vi "Collect information from UI to run measurement.vi"(8 "error in (no error)":errorcluster, 11 "Measurement UI in":refnum<class "Measurement UI.lvclass">) -> (0 "error out":errorcluster, 1 "Show UI?":bool, 2 "Device Names":string[](array[string]), 3 "Measurement UI out":refnum<class "Measurement UI.lvclass">, 4 "String":string, 5 "Measurement Name":string, 6 "Run continuously?":bool, 7 "Iterations":i32)   [LabVIEW 2017, in "Measurement UI.lvlib" / "Measurement UI.lvclass"]
uses:
  Measurement UI.lvclass
  Measurement UI.lvclass/Measurement UI.ctl
  Accessors/Read Measurement.vi
  Accessors/Read Power Supply.vi
  Accessors/Read Digitizer.vi
  Accessors/Read Function Generator.vi
  Read Multimeter.vi
  Accessors/Read Show FP_.vi
  Read Run Indefinitely.vi
  Accessors/Read Step Iterations.vi
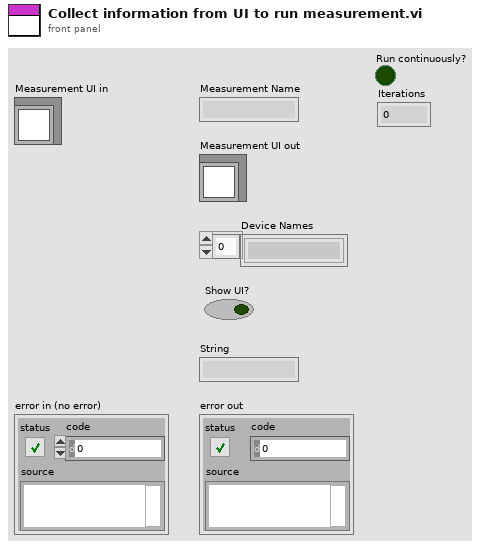
[diagram p1: front panel]
types:
  T1 = enum8{"Enabled", "Disabled", "Disabled and Grayed Out"}
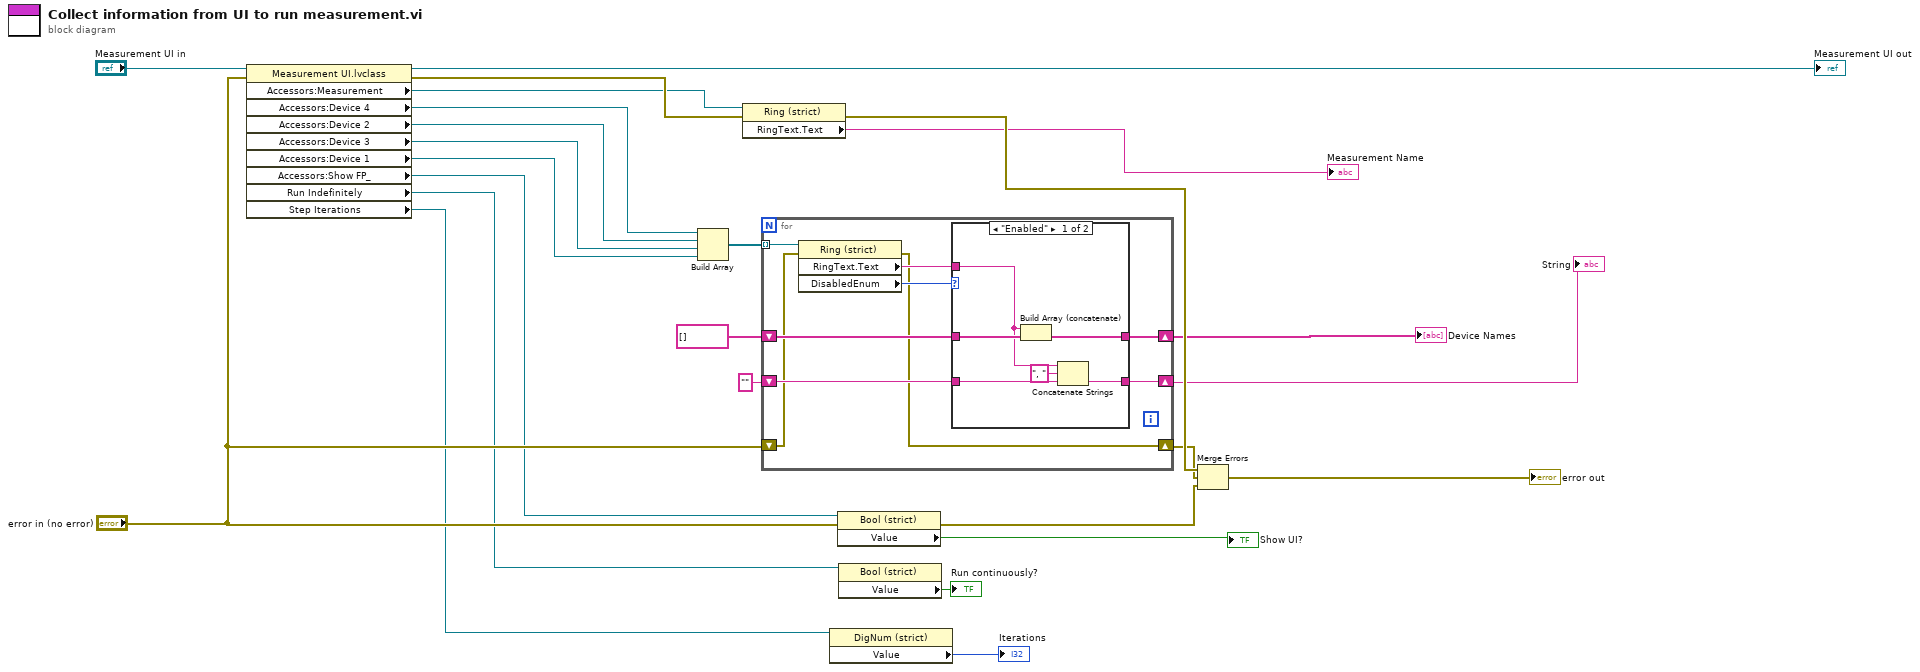
[diagram p0: block diagram]
diagram:
  n1 = property class="Measurement UI.lvclass"(reference="Measurement UI in", error in="error in (no error)") -> (reference out=→"Measurement UI out":refnum<class "Measurement UI.lvclass">, error out=w20:errorcluster, "Accessors:Measurement"=w19:refnum<vi>, "Accessors:Device 4"=w18:refnum<vi>, "Accessors:Device 2"=w17:refnum<vi>, "Accessors:Device 3"=w16:refnum<vi>, "Accessors:Device 1"=w15:refnum<vi>, "Accessors:Show FP_"=w14:refnum<vi>, "Run Indefinitely"=w4:refnum<vi>, "Step Iterations"=w2:refnum<vi>)
  n2 = Build Array(w18, w17, w16, w15) -> (w7:refnum<vi>[])
  n3 = property class="Ring (strict)"(reference=w19, error in=w20) -> (error out=w24:errorcluster, "RingText.Text"=→"Measurement Name":string)  [unwired: 1 out]
  n4 = for {
    shift-right: [w31] -> w6
    shift-left: string[] [] ("Device Names") -> [w30]
    tunnel: w7 -> [w34] mode=indexing
    shift-right: [w29] -> w11
    shift-left: "" -> [w28]
    shift-right: [w27] -> w22
    shift-left: "error in (no error)" -> [w26]
    n5 = property class="Ring (strict)"(reference=w34, error in=w26) -> (error out=w27:errorcluster, "RingText.Text"=w32:string, "DisabledEnum"=w33:T1)  [unwired: 1 out]
    n6 = case shown="\"Enabled\"" w33 {
      tunnel: w32 -> [w36 _]
      tunnel: [w40 w42] -> w31
      tunnel: w30 -> [w39 w42]
      tunnel: [w38 w41] -> w29
      tunnel: w28 -> [w37 w41]
      frame "Enabled" {
        n7 = Build Array (concatenate)(w36, w39) -> (w40:string[])
        n8 = Concatenate Strings(w36, ", " ("string"), w37) -> (w38:string)
      }
      frame "Disabled", Default {
      }
    }
  }
  "String" <- w11
  "Device Names" <- w6
  n9 = property class="DigNum (strict)"(reference=w2) -> ("Value"=→"Iterations":i32)  [unwired: 1 in, 2 out]
  n10 = property class="Bool (strict)"(reference=w14, error in="error in (no error)") -> (error out=w23:errorcluster, "Value"=→"Show UI?":bool)  [unwired: 1 out]
  n11 = property class="Bool (strict)"(reference=w4) -> ("Value"=→"Run continuously?":bool)  [unwired: 1 in, 2 out]
  n12 = Merge Errors(w24, w22, w23) -> (→"error out":errorcluster)
